vi "bar_code_reader.vi"() -> ()   [LabVIEW 2011]
uses:
  <vilib>/userDefined/High Color/IMAQdx.ctl
  <vilib>/vision/driver/IMAQdx.llb/IMAQdx Acquisition Mode.ctl
  <vilib>/vision/driver/IMAQdx.llb/IMAQdx Buffer Number Mode.ctl
  <vilib>/vision/driver/NI_Vision_Acquisition_Software.lvlib
panel:
  out "Image":T1(plugin-control)
  out "Acquisition Rate (frames/s)":dbl(knob) scale=0.0..110.0
  in  "stop":bool
  in  "Camera Name":T2
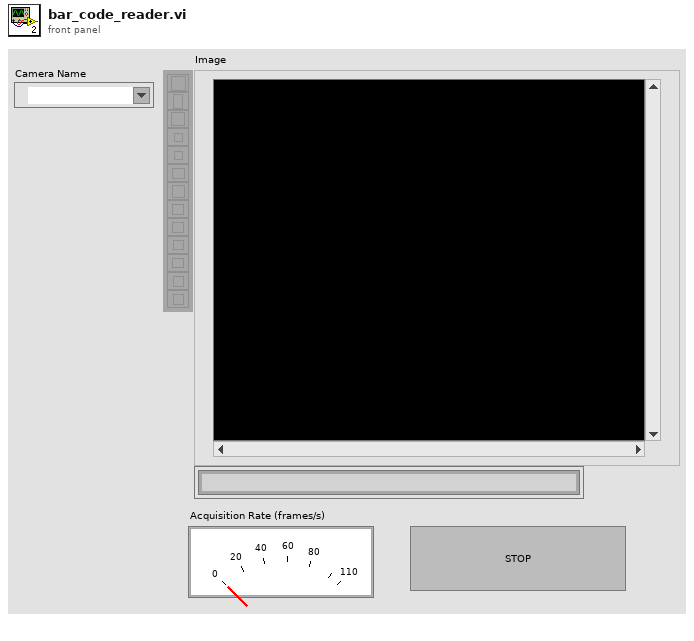
[diagram p1: front panel]
types:
  T1 = typedef "IMAQ Image.ctl" = refnum<image>
  T2 = typedef "IMAQdx.ctl" = refnum<k21>
  T3 = typedef "NI_Vision_Acquisition_Software.lvlib/IMAQdx Acquisition Mode.ctl" = enum32{"One Shot", "Continuous"}
  T4 = typedef "NI_Vision_Acquisition_Software.lvlib/IMAQdx Buffer Number Mode.ctl" = enum32{"Next", "Last", "Buffer Number"}
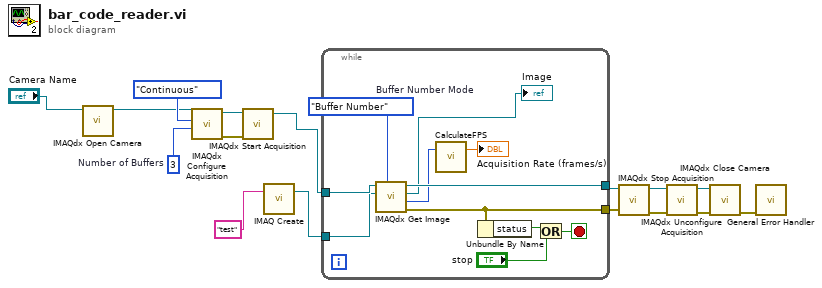
[diagram p0: block diagram]
diagram:
  w15 = u32 3  # Number of Buffers
  n1 = call <vilib>:"IMAQdx Open Camera.vi"("Session In"="Camera Name") -> ("Session Out"=w11:T2)  [unwired: 2 in, 8 out]
  n2 = call <vilib>:"IMAQdx Configure Acquisition.vi"("Number of Buffers"=w15, "Continuous?"=IMAQdx_Acquisition_Mode."Continuous", "Session In"=w11) -> ("error out"=w13:errorcluster, "Session Out"=w12:T2)  [unwired: 1 in, 6 out]
  n3 = call <vilib>:"IMAQdx Start Acquisition.vi"("error in"=w13, "Session In"=w12) -> ("Session Out"=w2:T2)  [unwired: 9 out]
  n4 = call "IMAQ Create"("Image Name"="test") -> ("New Image"=w1:T1)  [unwired: 3 in, 2 out]
  n5 = while {
    tunnel: [w25] -> w4
    tunnel: [w24] -> w3
    tunnel: w2 -> [w19]
    tunnel: w1 -> [w18]
    stop <- w27 stop-if-true
    w23 = IMAQdx_Buffer_Number_Mode."Buffer Number"  # Buffer Number Mode
    n6 = call <vilib>:"IMAQdx Get Image.vi"("Buffer Number Mode (Next)"=w23, "Image In"=w18, "Session In"=w19) -> ("error out"=w24:errorcluster, "Buffer Number Out"=w20:u32, "Image Out"=→"Image":T1, "Session Out"=w25:T2)  [unwired: 2 in, 3 out]
    n7 = call "CalculateFPS.vi"("buffer number"=w20) -> ("acquired FPS"=→"Acquisition Rate (frames/s)":dbl)  [unwired: 2 out]
    n8 = Unbundle By Name(w24) -> ("status"=w26:bool)
    n9 = Or(x=w26, y="stop") -> (x .or. y?=w27:bool)
  }
  n10 = call <vilib>:"IMAQdx Stop Acquisition.vi"("error in"=w3, "Session In"=w4) -> ("error out"=w5:errorcluster, "Session Out"=w6:T2)  [unwired: 8 out]
  n11 = call <vilib>:"IMAQdx Unconfigure Acquisition.vi"("error in"=w5, "Session In"=w6) -> ("error out"=w8:errorcluster, "Session Out"=w7:T2)  [unwired: 8 out]
  n12 = call <vilib>:"IMAQdx Close Camera.vi"("error in"=w8, "Session In"=w7) -> ("error out"=w9:errorcluster)  [unwired: 9 out]
  n13 = call <vilib>:"General Error Handler.vi"("error in (no error)"=w9) -> ()  [unwired: 1 in, 14 out]
